vi "Inverse_Kinematics(1).vi"(8 "L 2":dbl(slide)=115.0 scale=0.0..200.0, 9 "L 1":dbl(slide)=80.0 scale=0.0..200.0, 11 "end effector":cluster{dbl, dbl}={159.01647214211073, 1.9100783062530127} {"?" format="%.1f"; "?" format="%#.1f"}) -> (0 "Angle 2":dbl(knob)=-72.06882847083946 scale=-90.0..90.0, 1 "Angle1":dbl(knob)=-45.83837436417874 scale=-90.0..90.0)   [LabVIEW 2024]
panel:
  out "Animal Drawing":picture
  out "end effector 2":cluster{dbl, dbl}={159.01647214211073, 1.9100783062530127} {"?" format="%.1f"; "?" format="%#.1f"}
  out "2D Picture":picture
  # "mm"
  # "mm"
  # "mm"
  # "mm"
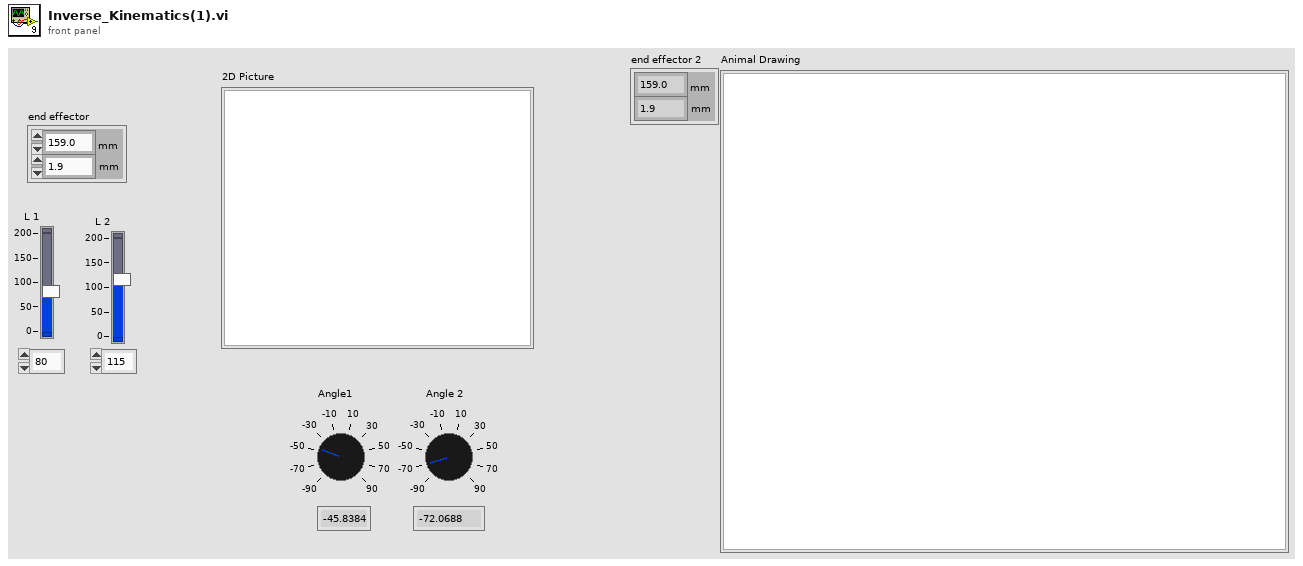
[diagram p1: front panel]
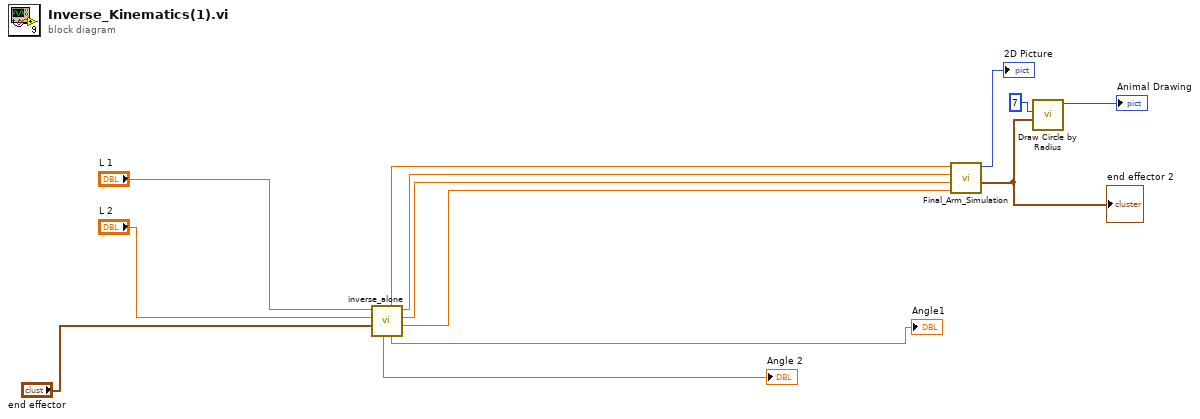
[diagram p0: block diagram]
diagram:
  n1 = call "inverse_alone.vi"("end effector"="end effector", "L in"="L 2", "L 1"="L 1") -> ("Numeric 2"=w11:dbl, "Numeric"=w5:dbl, "L 4"=w9:dbl, "Angle1"=→"Angle1":dbl, "L 3"=w8:dbl, "Angle 2"=→"Angle 2":dbl)  [unwired: 3 in]
  n2 = call "Final_Arm_Simulation.vi"("Angle 2"=w11, "Angle1"=w5, "L 2"=w9, "L 1"=w8) -> ("end effector"=w12:cluster{dbl, dbl}, "2D Picture"=→"2D Picture":picture)  [unwired: 6 in]
  "end effector 2" <- w12
  n3 = call <vilib>:"Draw Circle by Radius.vi"("pixel center"=w12, "radius"=i16 7) -> ("new picture"=→"Animal Drawing":picture)  [unwired: 9 in]
